vi "Calculate Required Steering Angle.vi"(7 "constraint error tolerance (1E-12)":dbl=1e-12, 8 "error in (no error)":errorcluster, 9 "wheel frame velocity":dbl[](array[numeric]), 11 "mecanum wheel in":refnum<class "NI_Robotics_Mecanum Wheel.lvclass">) -> (0 "error out":errorcluster, 2 "required steering angle (rad)":dbl, 3 "mecanum wheel out":refnum<class "NI_Robotics_Mecanum Wheel.lvclass">)   [LabVIEW 2017, in "NI_Robotics_Mecanum Wheel.lvclass"]
uses:
  <vilib>/robotics/Steering/Mecanum Wheel/NI_Robotics_Mecanum Wheel.lvclass
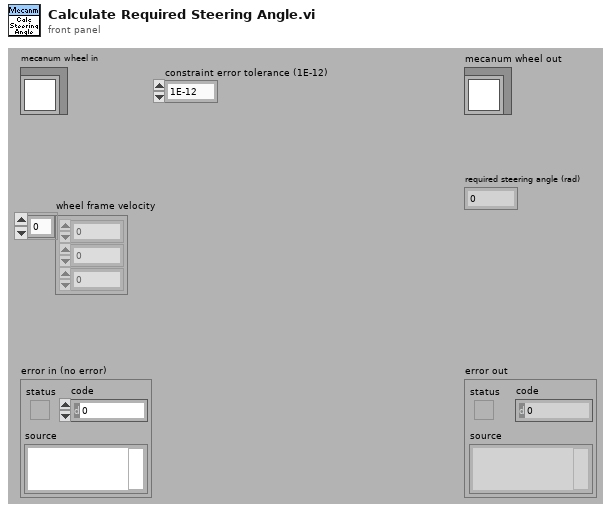
[diagram p1: front panel]
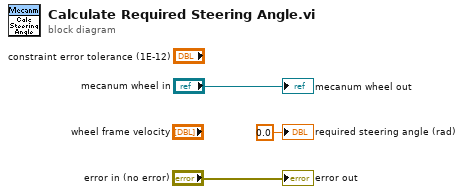
[diagram p0: block diagram]
diagram:
  "error out" <- "error in (no error)"
  "mecanum wheel out" <- "mecanum wheel in"
  "required steering angle (rad)" <- 0.0 ("Required Steering Angle")
